vi "Config - FGV.vi"(8 "Error In":errorcluster, 11 "Action":T2=enum."Get") -> (0 "Error Out":errorcluster, 3 "Out Cluster":T1={"Relative Array of paths"=["API", "Cfg", "Common", "Data", "Data\\Database_Script", "Data\\FW", "Data\\PIC", "Data\\DBC", "Data\\SSL_Certificates", "Debug", "Deployment", "Documentation", "Driver", "SEQ", "SEQ\\PreUUT\\Control", "SEQ\\PreUUT\\Module", "SEQ\\PreUUT\\Scanner", "SEQ\\CodeModule", "Tool", "Util"]})   [LabVIEW 2023, in "Abstraction_Interface.lvlib" / "Abstraction_Interface_Class.lvclass"]
uses:
  Abstraction_Interface_Class.lvclass
  Config - FGV - Action.ctl
  Config - Data Structure.ctl
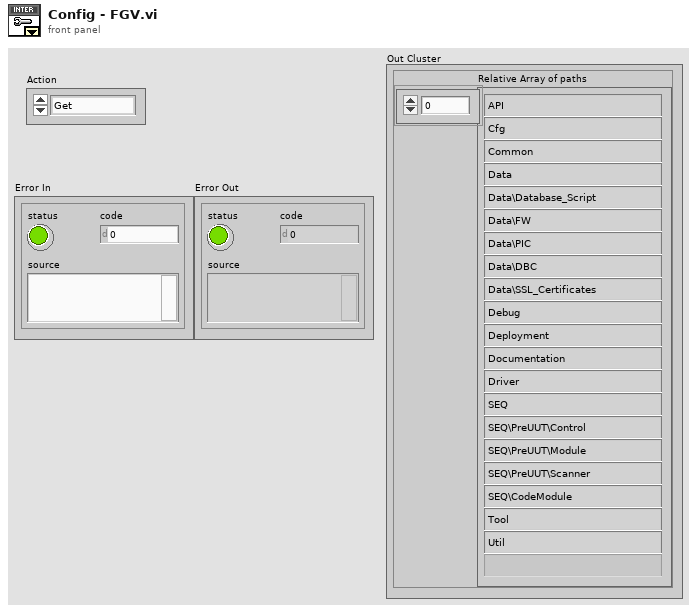
[diagram p1: front panel]
types:
  T1 = typedef "Abstraction_Interface.lvlib/Abstraction_Interface_Class.lvclass/Config - Data Structure.ctl" = cluster{"Relative Array of paths":string[]}
  T2 = typedef "Abstraction_Interface.lvlib/Abstraction_Interface_Class.lvclass/Config - FGV - Action.ctl" = enum16{"Init", "Get"}
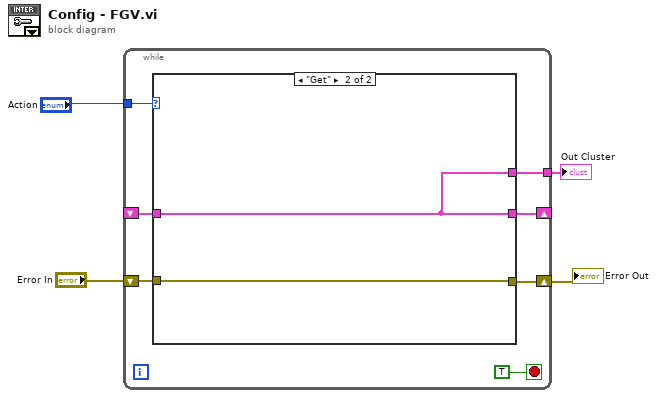
[diagram p0: block diagram]
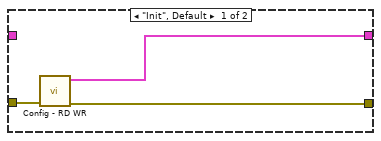
[diagram p2: hidden frame]
diagram:
  n1 = while {
    tunnel: "Action" -> [w10]
    shift-right: [w8] -> _
    shift-left: _ -> [w7]
    shift-right: [w6] -> w2
    shift-left: "Error In" -> [w9]
    tunnel: [w5] -> w1
    stop <- TRUE stop-if-true
    n2 = case shown="\"Get\"" w10 {
      tunnel: w9 -> [w14 w16]
      tunnel: [w13 w15] -> w8
      tunnel: w7 -> [_ w15]
      tunnel: [w12 w16] -> w6
      tunnel: [_ w15] -> w5
      frame "Init", Default {
        n3 = call "Config - RD WR.vi"("Error In"=w14) -> ("Error Out"=w12:errorcluster, "Out Cluster"=w13:T1)  [unwired: 9 in]
      }
      frame "Get" {
      }
    }
  }
  "Error Out" <- w2
  "Out Cluster" <- w1
